vi "Check_BSA_coms.vi"(7 "Multiply Velocity by -1":bool) -> (4 "Centre frequency":dbl format="%.2f", 5 "Bandwidth":dbl format="%.2f", 6 "Output":T4={"Output data format"=enum."Velocity", "Non-validated signals"=enum."Reject"}, 9 "Calibration factor":dbl=3.97 format="%.4f", 10 "Signal conditioning (out)":T5={"High voltage"=2000, "Signal gain (dB)"=45} {"Signal gain (dB)" min=0 max=57 step=1; "High voltage" min=0 max=2040 step=8}, 11 "Buffer mode out":enum16{"One shot", "Ring", "FIFO"}(ring), 12 "Anode current limit (mA)":T7(ring), 14 "Range (out)":T6={"Centre frequency"=16, "Bandwidth"=10, "Units"=enum."m/s", "Frequency shift"=enum."Enabled"} {"Bandwidth" items=["3.776E-3", "7.553E-3", "15.105E-3", "30.211E-3", "60.422E-3", "120.844E-3", "241.687E-3", "483.375E-3", "966.750E-3", "1.933E+0", "3.867E+0", "7.734E+0", "15.468E+0", "30.936E+0"]; "Centre frequency" items=["-15.468E+0", "-14.501E+0", "-13.534E+0", "-12.568E+0", "-11.601E+0", "-10.634E+0", "-9.667E+0", "-8.701E+0", "-7.734E+0", "-6.767E+0", "-5.800E+0", "-4.834E+0", "-3.867E+0", "-2.900E+0", "-1.933E+0", "-966.750E-3", "0.000E+0", "966.750E-3", "1.933E+0", "2.900E+0", "3.867E+0", "4.834E+0", "5.800E+0", "6.767E+0", "7.734E+0", "8.701E+0", "9.667E+0", "10.634E+0", "11.601E+0", "12.568E+0", "13.534E+0", "14.501E+0", "15.468E+0"]}, 15 "Selected range":cluster{"Minimum":dbl, "Maximum":dbl}={"Minimum"=-1.9850000000000005, "Maximum"=1.9850000000000005} {"Maximum" format="%.2f"; "Minimum" format="%.2f"}, 17 "Clock parameters (out)":T1={"Arrival time clock"=enum."Internal", "Clock source"=enum."Private", "Coincidence"=enum."Master"}, 18 "Data collection mode (out)":T3 {"Duty cycle (%)" format="%.2f"; "Dead time (s)" format="%.2f"}, 19 "Analysis parameters (out)":T2={"Burst criterion"=enum."Envelope", "Oversize reject level"=enum."1 (disabled)", "Pedestal attenuation"=enum."0", "Record length"=enum."16", "Quality factor"=0} {"Quality factor" min=0 max=80 step=10})   [LabVIEW 2010]
uses:
  Anemometry Sub Vis/Controls/ok_button.ctl
panel:
  in  "Wavelength (nm)":dbl=514.5 format="%.1f"
  in  "GPIB Address":string="13"
  in  "Focal Length (mm)":dbl=50.0
  in  "Beam Separation (mm)":dbl=8.0
  out "Read Setup string":string
  out "error out":errorcluster
  in  "Clock parameters":T1={"Arrival time clock"=enum."Internal", "Clock source"=enum."Private", "Coincidence"=enum."Master"}
  in  "Analysis parameters":T2={"Burst criterion"=enum."Envelope", "Oversize reject level"=enum."1 (disabled)", "Pedestal attenuation"=enum."0", "Record length"=enum."16", "Quality factor"=0} {"Quality factor" min=0 max=80 step=10}
  in  "Data collection mode":T3 {"Duty cycle (%)" format="%.2f"; "Dead time (s)" format="%.2f"}
  in  "Buffer mode":enum16{"One shot", "Ring", "FIFO"}(ring)
  in  "OK":T8
  in  "Signal conditioning":T5={"High voltage"=1600, "Signal gain (dB)"=35} {"Signal gain (dB)" min=0 max=57 step=1; "High voltage" min=0 max=1600 step=8}
  in  "Range":T9={"Centre Velocity"=16, "Velocity span"=10, "Units"=enum."m/s", "Frequency shift"=enum."Enabled"} {"Velocity span" items=["3.582E-3", "7.164E-3", "14.328E-3", "28.656E-3", "57.312E-3", "114.625E-3", "229.250E-3", "458.500E-3", "917.000E-3", "1.834E+0", "3.668E+0", "7.336E+0", "14.672E+0", "29.344E+0"]; "Centre Velocity" items=["-7.336E+0", "-6.877E+0", "-6.419E+0", "-5.960E+0", "-5.502E+0", "-5.043E+0", "-4.585E+0", "-4.127E+0", "-3.668E+0", "-3.209E+0", "-2.751E+0", "-2.292E+0", "-1.834E+0", "-1.375E+0", "-917.000E-3", "-458.500E-3", "0.000E+0", "458.500E-3", "917.000E-3", "1.375E+0", "1.834E+0", "2.292E+0", "2.751E+0", "3.209E+0", "3.668E+0", "4.127E+0", "4.585E+0", "5.043E+0", "5.502E+0", "5.960E+0", "6.419E+0", "6.877E+0", "7.336E+0"]}
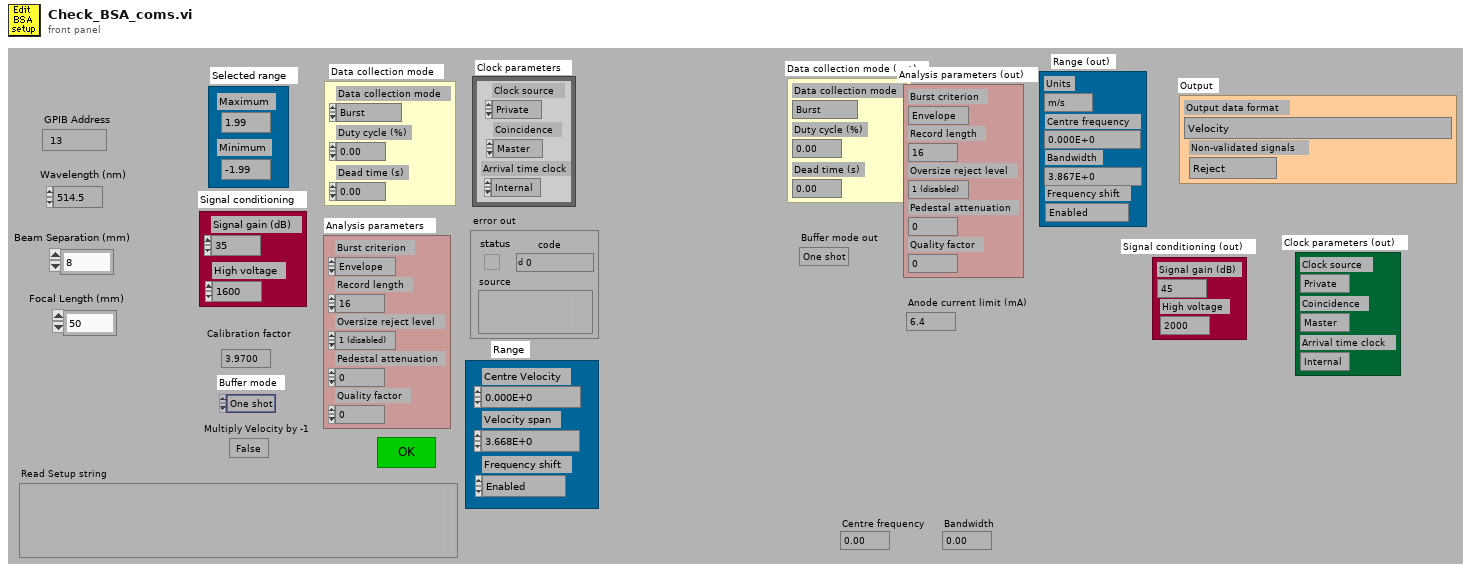
[diagram p1: front panel]
types:
  T1 = cluster{"Arrival time clock":enum16{"External", "Internal"}, "Clock source":enum16{"Slave", "Master", "Private"}, "Coincidence":enum16{"Slave", "Master", "Private"}}
  T2 = cluster{"Burst criterion":enum16{"Envelope", "Pedestal", "Env and ped"}, "Oversize reject level":enum16{"1 (disabled)", "2", "3", "4", "5", "6", "7", "8", "9"}, "Pedestal attenuation":enum16{"0", "6", "12", "18"}, "Record length":enum16{"8", "16", "32", "64"}, "Quality factor":i16}
  T3 = cluster{"Dead time (s)":dbl, "Duty cycle (%)":dbl, "Data collection mode":enum16{"Burst", "Contiuous", "Dead time", "External"}}
  T4 = cluster{"Output data format":enum16{"Velocity, transit time, arrival time", "Velocity, arrival time", "Velocity, transit time", "Velocity"}, "Non-validated signals":enum16{"Accept", "Reject"}}
  T5 = cluster{"High voltage":i16, "Signal gain (dB)":i16}
  T6 = cluster{"Centre frequency":u16, "Bandwidth":u16, "Units":enum16{"Hz", "m/s"}, "Frequency shift":enum16{"Disabled", "Enabled"}}
  T7 = enum16{"6.4", "3.2", "1.6", "0.8", "0.4", "0.2", "0.1", "0.05"}
  T8 = typedef "ok_button.ctl" = bool
  T9 = cluster{"Centre Velocity":u16, "Velocity span":u16, "Units":enum16{"Hz", "m/s"}, "Frequency shift":enum16{"Disabled", "Enabled"}}
  T10 = enum16{"Burst", "Contiuous", "Dead time", "External"}
  T11 = enum16{"1 (disabled)", "2", "3", "4", "5", "6", "7", "8", "9"}
  T12 = enum16{"Velocity, transit time, arrival time", "Velocity, arrival time", "Velocity, transit time", "Velocity"}
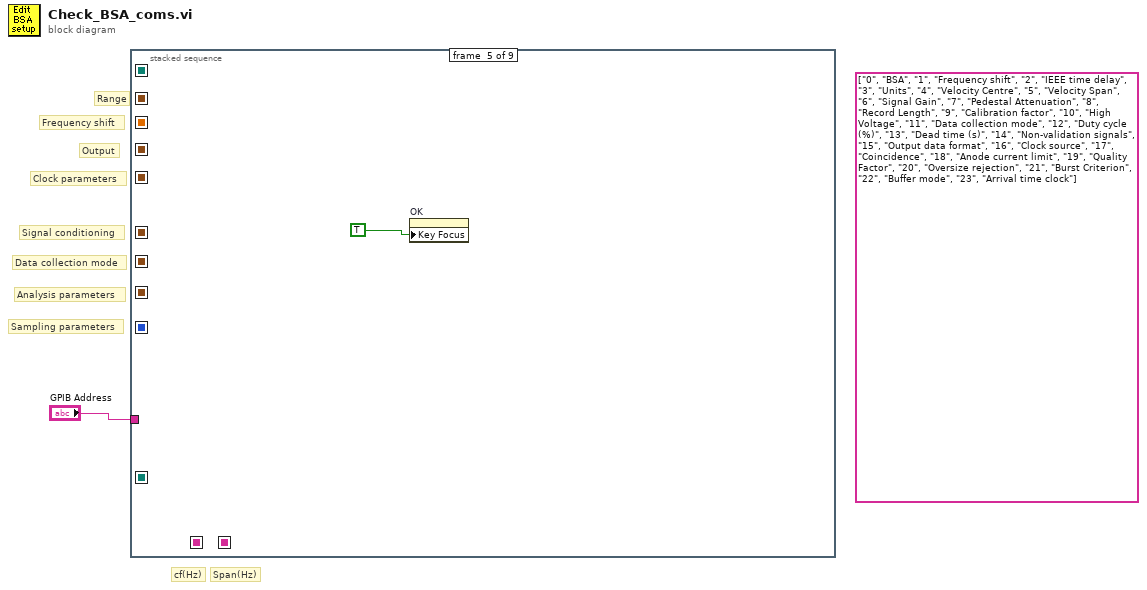
[diagram p0: block diagram]
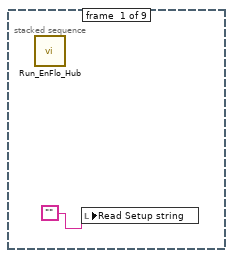
[diagram p2: hidden frame]
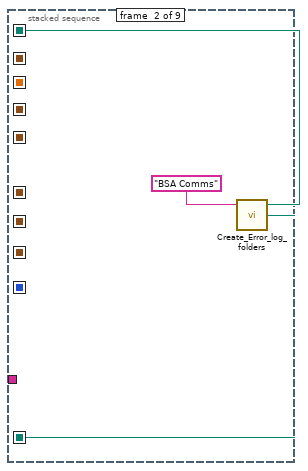
[diagram p3: hidden frame]
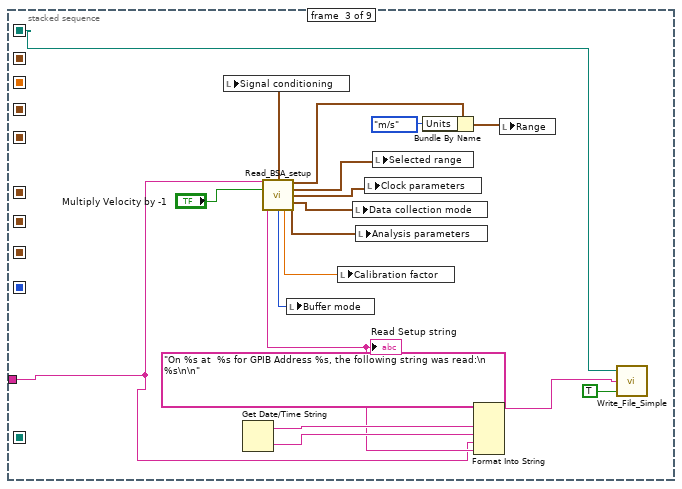
[diagram p4: hidden frame]
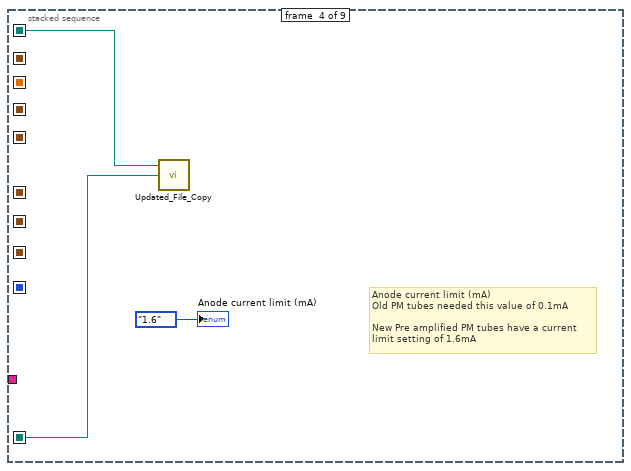
[diagram p5: hidden frame]
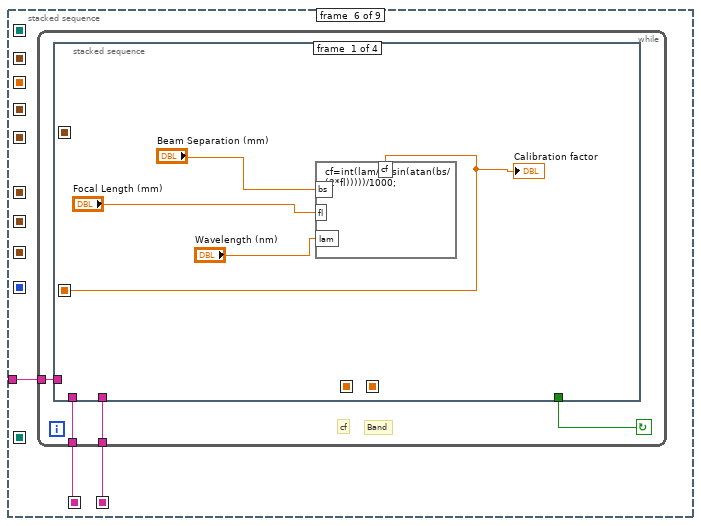
[diagram p6: hidden frame]
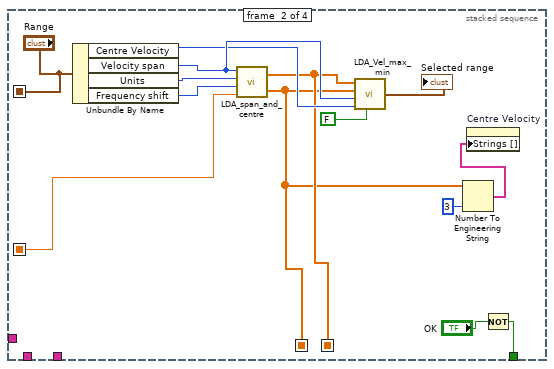
[diagram p7: hidden frame]
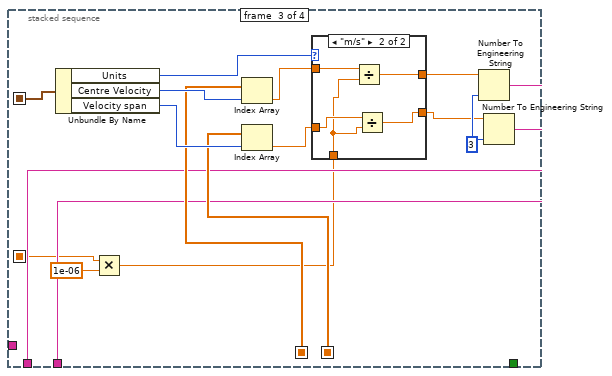
[diagram p8: hidden frame]
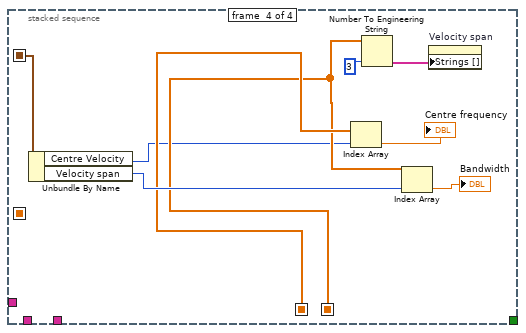
[diagram p10: hidden frame]
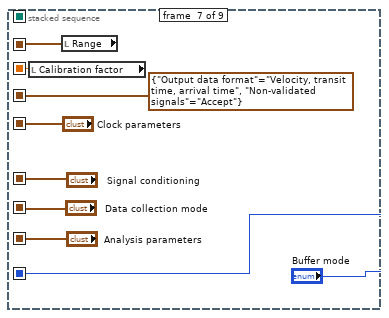
[diagram p11: hidden frame]
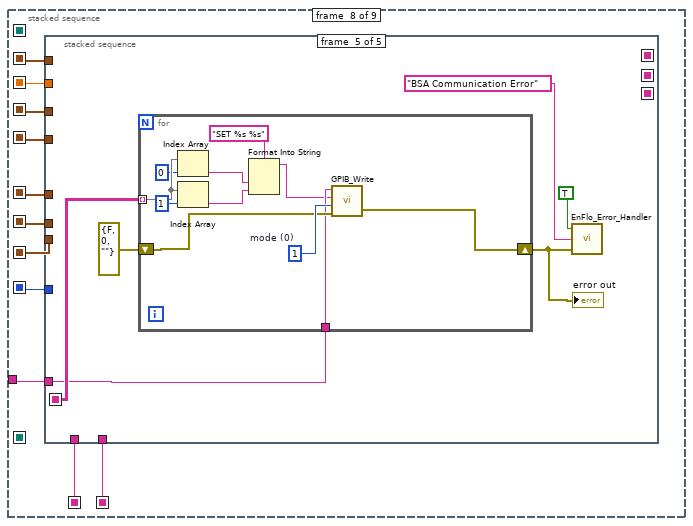
[diagram p12: hidden frame]
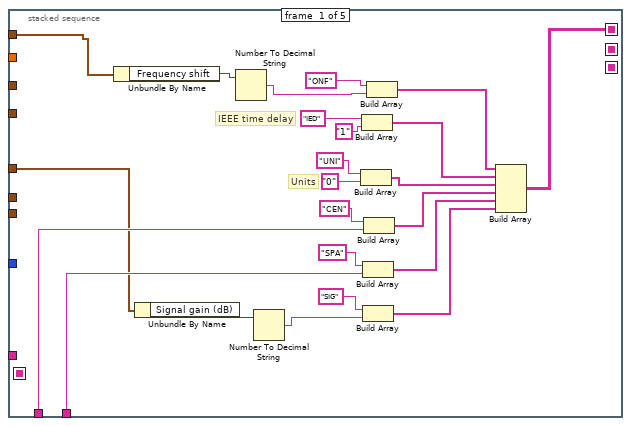
[diagram p13: hidden frame]
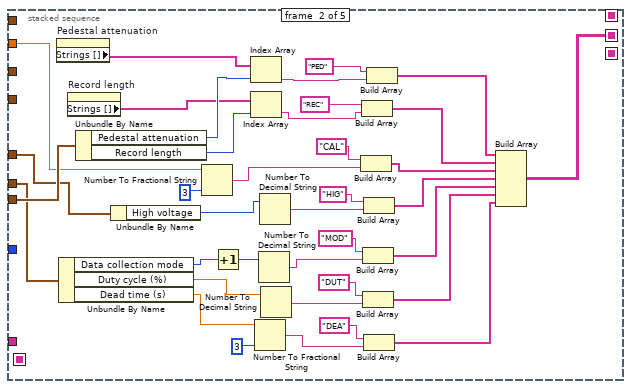
[diagram p14: hidden frame]
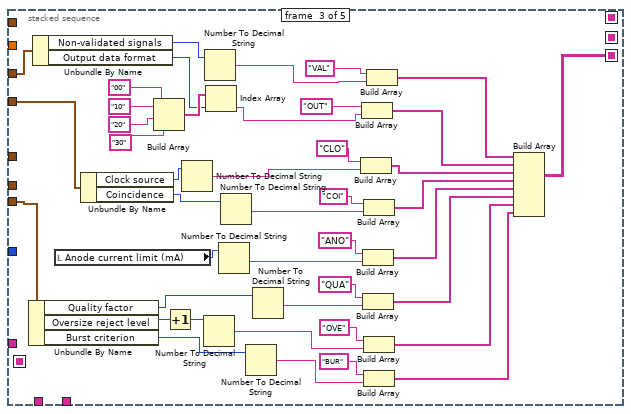
[diagram p15: hidden frame]
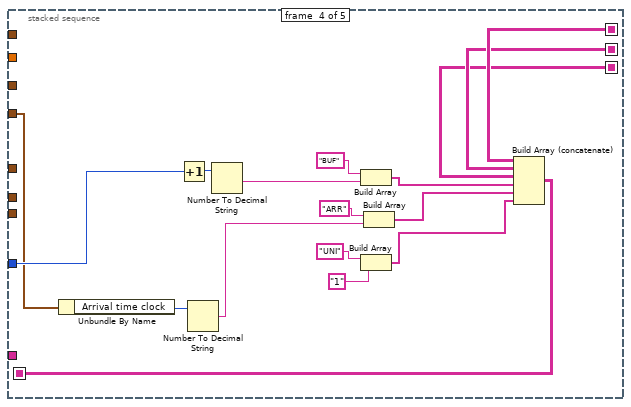
[diagram p16: hidden frame]
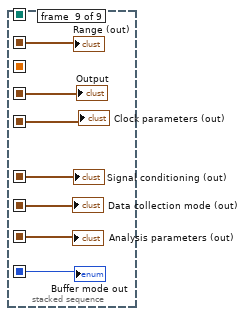
[diagram p17: hidden frame]
diagram:
  (unwired) string[][] [["0", "BSA"], ["1", "Frequency shift"], ["2", "IEEE time delay"], ["3", "Units"], ["4", "Velocity Centre"], ["5", "Velocity Span"], ["6", "Signal Gain"], ["7", "Pedestal Attenuation"], ["8", "Record Length"], ["9", "Calibration factor"], ["10", "High Voltage"], ["11", "Data collection mode"], ["12", "Duty cycle (%)"], ["13", "Dead time (s)"], ["14", "Non-validation signals"], ["15", "Output data format"], ["16", "Clock source"], ["17", "Coincidence"], ["18", "Anode current limit"], ["19", "Quality Factor"], ["20", "Oversize rejection"], ["21", "Burst Criterion"], ["22", "Buffer mode"], ["23", "Arrival time clock"]]
  # "Span(Hz)"
  # "cf(Hz)"
  # "Sampling parameters"
  # "Clock parameters"
  # "Output"
  # "Frequency shift"
  # "Data collection mode"
  # "Analysis parameters"
  # "Signal conditioning"
  # "Range"
  n1 = stacked-sequence {
    seq-local: [_ _ _ _ _ _ w90 _ _] -> [_ _ _ _ _ _ _ w104 w247]
    seq-local: [_ _ _ _ _ _ w91 _ _] -> [_ _ _ _ _ _ _ w103 _]
    seq-local: [_ _ _ _ _ _ T4 {"Output data format"=enum."Velocity, transit time, arrival time", "Non-validated signals"=enum."Accept"} ("Output") _ _] -> [_ _ _ _ _ _ _ w102 w242]
    seq-local: [_ _ _ _ _ _ "Clock parameters" _ _] -> [_ _ _ _ _ _ _ w101 w243]
    seq-local: [_ _ _ _ _ _ "Signal conditioning" _ _] -> [_ _ _ _ _ _ _ w100 w244]
    seq-local: [_ _ _ _ _ _ "Data collection mode" _ _] -> [_ _ _ _ _ _ _ w99 w246]
    seq-local: [_ _ _ _ _ _ "Analysis parameters" _ _] -> [_ _ _ _ _ _ _ w98 w245]
    seq-local: [_ _ _ _ _ _ "Buffer mode" _ _] -> [_ _ _ _ _ _ _ w97 w241]
    seq-local: [_ _ _ _ _ w31 _ _ _] -> [_ _ _ _ _ _ _ w95 _]
    seq-local: [_ _ _ _ _ w30 _ _ _] -> [_ _ _ _ _ _ _ w94 _]
    seq-local: [_ w4 _ _ _ _ _ _ _] -> [_ _ w7 w26 _ _ _ _ _]
    seq-local: [_ w3 _ _ _ _ _ _ _] -> [_ _ _ w25 _ _ _ _ _]
    tunnel: "GPIB Address" -> [_ _ w9 _ _ w29 _ w96 _]
    frame #0 {
      n2 = call "Run_EnFlo_Hub.vi"() -> ()  [unwired: 8 in]
      n3 = local write "Read Setup string"("") -> ()
    }
    frame #1 {
      n4 = call "Create_Error_log_folders.vi"("Log Filename"="BSA Comms" ("Input Element")) -> ("Server copy Location"=w3:path, "Local Log File"=w4:path)  [unwired: 2 in, 1 out]
    }
    frame #2 {
      n5 = Get Date/Time String() -> (date string=w13:string, time string=w12:string)  [unwired: 3 in]
      n6 = call "Read_BSA_setup.vi"("GPIB Address"=w9, "Multiply Velocity by -1"="Multiply Velocity by -1") -> ("Signal conditioning"=w24:T5, "Range"=w17:T9, "Selected range"=w18:cluster{"Minimum":dbl, "Maximum":dbl}, "Clock parameters"=w19:T1, "Data collection mode"=w20:T3, "Setup string"=w11:string, "Buffer mode"=w23:enum16{"One shot", "Ring", "FIFO"}, "Calibration factor"=w22:dbl, "Analysis parameters"=w21:T2)  [unwired: 1 in, 4 out]
      "Read Setup string" <- w11
      n7 = local write "Signal conditioning"(w24) -> ()
      n8 = local write "Buffer mode"(w23) -> ()
      n9 = local write "Calibration factor"(w22) -> ()
      n10 = local write "Data collection mode"(w20) -> ()
      n11 = local write "Analysis parameters"(w21) -> ()
      n12 = local write "Clock parameters"(w19) -> ()
      n13 = local write "Selected range"(w18) -> ()
      n14 = Bundle By Name(cluster=w17, "Units"=enum16{"Hz", "m/s"}."m/s") -> (w16:T9)
      n15 = Format Into String(format string="On %s at  %s for GPIB Address %s, the following string was read:\n %s\n\n", w13, w12, w9, w11) -> (resulting string=w6:string)  [unwired: 2 in, 1 out]
      n16 = local write "Range"(w16) -> ()
      n17 = call "Write_File_Simple.vi"("append to file? (new file:F)"=TRUE, "character string"=w6, "file path"=w7) -> ()  [unwired: 2 out]
    }
    frame #3 {
      # "Anode current limit (mA)\nOld PM tubes needed this value of 0.1mA\n\nNew Pre amplified PM tubes have a current\nlimit setting of 1.6mA"
      n18 = call "Updated_File_Copy.vi"("Target Path"=w25, "Source Path"=w26) -> ()  [unwired: 1 in, 1 out]
      "Anode current limit (mA)" <- T7."1.6" ("Anode current limit (mA)")
    }
    frame #4 {
      n19 = property on="OK" class="Bool"("Key Focus"=TRUE ("Visible")) -> ()  [unwired: 2 in, 2 out]
    }
    frame #5 {
      n20 = while {
        tunnel: [w33] -> w30
        tunnel: [w34] -> w31
        tunnel: w29 -> [w32]
        stop <- w35 continue-if-true
        # "Band"
        # "cf"
        n21 = stacked-sequence {
          seq-local: [w39 _ _ _] -> [_ w41 w61 _]
          seq-local: [_ w42 _ _] -> [_ _ w65 w81]
          seq-local: [_ w45 _ _] -> [_ _ w64 w80]
          seq-local: [_ "Range" _ _] -> [_ _ w69 w85]
          tunnel: [_ w52 _ _] -> w35
          tunnel: [_ _ w63 _] -> w34
          tunnel: [_ _ w62 _] -> w33
          tunnel: w32 -> [_ _ _ _]
          frame #0 {
            n22 = formula code="cf=int(lam/2/(sin(atan(bs/(2*fl)))))/1000;"("bs"="Beam Separation (mm)", "fl"="Focal Length (mm)", "lam"="Wavelength (nm)") -> ("cf"=w39:dbl)
            "Calibration factor" <- w39
          }
          frame #1 {
            n23 = Unbundle By Name("Range") -> ("Centre Velocity"=w47:u16, "Velocity span"=w48:u16, "Units"=w50:enum16{"Hz", "m/s"}, "Frequency shift"=w49:enum16{"Disabled", "Enabled"})
            n24 = call "LDA_span_and_centre.vi"("Calibration factor"=w41, "Frequency shift"=w49, "Units"=w50, "Velocity span"=w48) -> ("Centres"=w42:dbl[], "Spans"=w45:dbl[])
            n25 = call "LDA_Vel_max_min.vi"("Multiply Velocity by -1"=FALSE, "Centre Velocity"=w47, "Velocity span"=w48, "Centres"=w42, "Spans"=w45) -> ("Selected range"=→"Selected range":cluster{"Minimum":dbl, "Maximum":dbl})  [unwired: 1 in]
            n26 = Number To Engineering String(2:i16 3 ("precision (6)"), 4:w42) -> (0:w43:string[])  [unwired: 2 in]
            n27 = property on="Centre Velocity" class="Ring (strict)"("Strings []"=w43) -> ()  [unwired: 2 in, 2 out]
            n28 = Not(x="OK") -> (.not. x?=w52:T8)
          }
          frame #2 {
            w66 = 3
            n29 = Unbundle By Name(w69) -> ("Units"=w56:enum16{"Hz", "m/s"}, "Centre Velocity"=w67:u16, "Velocity span"=w68:u16)
            n30 = Multiply(x=w61, y=1e-06) -> (x*y=w59:dbl)
            n31 = Index Array(array=w65, index=w67) -> (element=w57:dbl)
            n32 = Index Array(array=w64, index=w68) -> (element=w58:dbl)
            n33 = case shown="\"m/s\"" w56 {
              tunnel: w57 -> [w71 w76]
              tunnel: [w71 w72] -> w55
              tunnel: w58 -> [w70 w75]
              tunnel: [w70 w73] -> w54
              tunnel: w59 -> [_ w74]
              frame "Hz" {
              }
              frame "m/s" {
                n34 = Divide(x=w76, y=w74) -> (x/y=w72:dbl)
                n35 = Divide(x=w75, y=w74) -> (x/y=w73:dbl)
              }
            }
            n36 = Number To Engineering String(2:w66, 4:w55) -> (0:w63:string)  [unwired: 2 in]
            n37 = Number To Engineering String(2:w66, 4:w54) -> (0:w62:string)  [unwired: 2 in]
          }
          frame #3 {
            n38 = Unbundle By Name(w85) -> ("Centre Velocity"=w78:u16, "Velocity span"=w82:u16)
            n39 = Index Array(array=w81, index=w78) -> (element=→"Centre frequency":dbl)
            n40 = Number To Engineering String(2:3, 4:w80) -> (0:w79:string[])  [unwired: 2 in]
            n41 = Index Array(array=w80, index=w82) -> (element=→"Bandwidth":dbl)
            n42 = property on="Velocity span" class="Ring (strict)"("Strings []"=w79) -> ()  [unwired: 2 in, 2 out]
          }
        }
      }
    }
    frame #6 {
      n43 = local read "Calibration factor"() -> (w91:dbl)
      n44 = local read "Range"() -> (w90:T9)
    }
    frame #7 {
      n45 = stacked-sequence {
        seq-local: [w105 _ _ _ _] -> [_ _ _ w213 _]
        seq-local: [_ w130 _ _ _] -> [_ _ _ w212 _]
        seq-local: [_ _ w166 _ _] -> [_ _ _ w211 _]
        seq-local: [_ _ _ w210 _] -> [_ _ _ _ w229]
        tunnel: w104 -> [w127 _ _ _ _]
        tunnel: w95 -> [w118 _ _ _ _]
        tunnel: w94 -> [w116 _ _ _ _]
        tunnel: w100 -> [w113 w144 _ _ _]
        tunnel: w98 -> [_ w152 w175 _ _]
        tunnel: w103 -> [_ w146 _ _ _]
        tunnel: w99 -> [_ w141 _ _ _]
        tunnel: w102 -> [_ _ w192 _ _]
        tunnel: w101 -> [_ _ w182 w216 _]
        tunnel: w97 -> [_ _ _ w218 _]
        tunnel: w96 -> [_ _ _ _ w224]
        frame #0 {
          # "Units"
          # "IEEE time delay"
          n46 = Unbundle By Name(w127) -> ("Frequency shift"=w126:enum16{"Disabled", "Enabled"})
          n47 = Unbundle By Name(w113) -> ("Signal gain (dB)"=w114:i16)
          n48 = Number To Decimal String(number=w126) -> (decimal integer string=w124:string)  [unwired: 1 in]
          n49 = Number To Decimal String(number=w114) -> (decimal integer string=w112:string)  [unwired: 1 in]
          n50 = Build Array("UNI", "0") -> (w109:string[])
          n51 = Build Array("IED", "1" ("element")) -> (w110:string[])
          n52 = Build Array("SPA", w116) -> (w107:string[])
          n53 = Build Array("SIG", w112) -> (w106:string[])
          n54 = Build Array("CEN", w118) -> (w108:string[])
          n55 = Build Array("ONF", w124) -> (w111:string[])
          n56 = Build Array(w111, w110, w109, w108, w107, w106) -> (w105:string[][])
        }
        frame #1 {
          n57 = property on="Pedestal attenuation" class="Enum (strict)"() -> ("Strings []"=w129:string[])  [unwired: 2 in, 2 out]
          n58 = Unbundle By Name(w141) -> ("Data collection mode"=w136:T10, "Duty cycle (%)"=w135:dbl, "Dead time (s)"=w134:dbl)
          n59 = property on="Record length" class="Enum (strict)"() -> ("Strings []"=w128:string[])  [unwired: 2 in, 2 out]
          n60 = Unbundle By Name(w152) -> ("Pedestal attenuation"=w151:enum16{"0", "6", "12", "18"}, "Record length"=w150:enum16{"8", "16", "32", "64"})
          n61 = Unbundle By Name(w144) -> ("High voltage"=w143:i16)
          n62 = Number To Fractional String(number=w146, precision (6)=3) -> (F-format string=w145:string)  [unwired: 2 in]
          n63 = Increment(x=w136) -> (x+1=w139:T10)
          n64 = Index Array(array=w129, index=w151) -> (element=w148:string)
          n65 = Index Array(array=w128, index=w150) -> (element=w149:string)
          n66 = Number To Fractional String(number=w134, precision (6)=3) -> (F-format string=w133:string)  [unwired: 2 in]
          n67 = Number To Decimal String(number=w139) -> (decimal integer string=w131:string)  [unwired: 1 in]
          n68 = Number To Decimal String(number=w143) -> (decimal integer string=w142:string)  [unwired: 1 in]
          n69 = Number To Decimal String(number=w135) -> (decimal integer string=w132:string)  [unwired: 1 in]
          n70 = Build Array("CAL", w145) -> (w156:string[])
          n71 = Build Array("REC", w149) -> (w157:string[])
          n72 = Build Array("MOD", w131) -> (w154:string[])
          n73 = Build Array("DUT", w132) -> (w153:string[])
          n74 = Build Array("HIG", w142) -> (w155:string[])
          n75 = Build Array("DEA", w133) -> (w137:string[])
          n76 = Build Array("PED", w148) -> (w158:string[])
          n77 = Build Array(w158, w157, w156, w155, w154, w153, w137) -> (w130:string[][])
        }
        frame #2 {
          n78 = Unbundle By Name(w175) -> ("Quality factor"=w173:i16, "Oversize reject level"=w172:T11, "Burst criterion"=w171:enum16{"Envelope", "Pedestal", "Env and ped"})
          n79 = Unbundle By Name(w192) -> ("Non-validated signals"=w186:enum16{"Accept", "Reject"}, "Output data format"=w185:T12)
          n80 = local read "Anode current limit (mA)"() -> (w165:T7)
          n81 = Unbundle By Name(w182) -> ("Clock source"=w181:enum16{"Slave", "Master", "Private"}, "Coincidence"=w180:enum16{"Slave", "Master", "Private"})
          n82 = Build Array("00", "10", "20", "30") -> (w187:string[])
          n83 = Increment(x=w172) -> (x+1=w174:T11)
          n84 = Number To Decimal String(number=w181) -> (decimal integer string=w179:string)  [unwired: 1 in]
          n85 = Number To Decimal String(number=w174) -> (decimal integer string=w169:string)  [unwired: 1 in]
          n86 = Number To Decimal String(number=w186) -> (decimal integer string=w184:string)  [unwired: 1 in]
          n87 = Index Array(array=w187, index=w185) -> (element=w183:string)
          n88 = Number To Decimal String(number=w165) -> (decimal integer string=w177:string)  [unwired: 1 in]
          n89 = Number To Decimal String(number=w180) -> (decimal integer string=w178:string)  [unwired: 1 in]
          n90 = Number To Decimal String(number=w171) -> (decimal integer string=w170:string)  [unwired: 1 in]
          n91 = Number To Decimal String(number=w173) -> (decimal integer string=w168:string)  [unwired: 1 in]
          n92 = Build Array("CLO", w179) -> (w198:string[])
          n93 = Build Array("OUT", w183) -> (w199:string[])
          n94 = Build Array("ANO", w177) -> (w196:string[])
          n95 = Build Array("QUA", w168) -> (w195:string[])
          n96 = Build Array("COI", w178) -> (w197:string[])
          n97 = Build Array("OVE", w169) -> (w193:string[])
          n98 = Build Array("BUR", w170) -> (w167:string[])
          n99 = Build Array("VAL", w184) -> (w200:string[])
          n100 = Build Array(w200, w199, w198, w197, w196, w195, w193, w167) -> (w166:string[][])
        }
        frame #3 {
          n101 = Unbundle By Name(w216) -> ("Arrival time clock"=w215:enum16{"External", "Internal"})
          n102 = Increment(x=w218) -> (x+1=w219:enum16{"One shot", "Ring", "FIFO"})
          n103 = Number To Decimal String(number=w215) -> (decimal integer string=w214:string)  [unwired: 1 in]
          n104 = Number To Decimal String(number=w219) -> (decimal integer string=w217:string)  [unwired: 1 in]
          n105 = Build Array("BUF", w217) -> (w221:string[])
          n106 = Build Array("UNI", "1" ("element")) -> (w207:string[])
          n107 = Build Array("ARR", w214) -> (w220:string[])
          n108 = Build Array (concatenate)(w213, w212, w211, w221, w220, w207) -> (w210:string[][])
        }
        frame #4 {
          n109 = for {
            tunnel: w229 -> [w236] mode=indexing
            shift-right: [w239] -> w225
            shift-left: errorcluster {"status"=FALSE, "code"=0, "source"=""} ("error out") -> [w238]
            tunnel: w224 -> [w237]
            w240 = i16 1  # mode (0)
            n110 = Index Array(array=w236, index=0) -> (element=w233:string)
            n111 = Index Array(array=w236, index=1) -> (element=w232:string)
            n112 = Format Into String(format string="SET %s %s", w233, w232) -> (resulting string=w230:string)  [unwired: 2 in, 1 out]
            n113 = call "GPIB_Write.vi"("address string"=w237, "data In"=w230, "mode (0)"=w240, "error in"=w238) -> ("error out"=w239:errorcluster)  [unwired: 1 in, 1 out]
          }
          "error out" <- w225
          n114 = call "EnFlo_Error_Handler.vi"("error in (no error)"=w225, "Error Type"="BSA Communication Error", "Dialog Box (T)"=TRUE) -> ()  [unwired: 3 out]
        }
      }
    }
    frame #8 {
      "Range (out)" <- w247
      "Signal conditioning (out)" <- w244
      "Analysis parameters (out)" <- w245
      "Output" <- w242
      "Clock parameters (out)" <- w243
      "Data collection mode (out)" <- w246
      "Buffer mode out" <- w241
    }
  }
